vi "Initialize_measurement.vi"(8 "Measurement":string, 9 "Spectrum Only?":bool, 11 "file path":path) -> (0 "error out":errorcluster, 1 "Group Name":string, 3 "tdms file out":refnum<k34>)   [LabVIEW 2019]
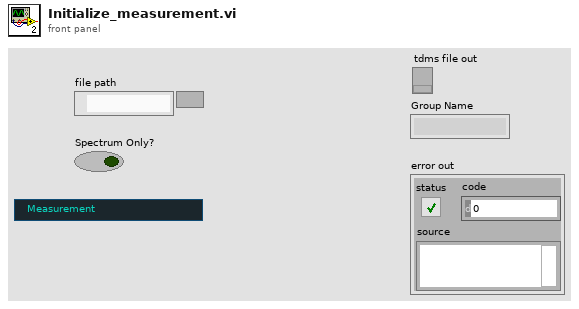
[diagram p1: front panel]
types:
  T1 = enum16{"big-endian, network order", "native, host order", "little-endian"}
  T2 = enum16{"open", "open or create", "create or replace", "create", "open (read-only)"}
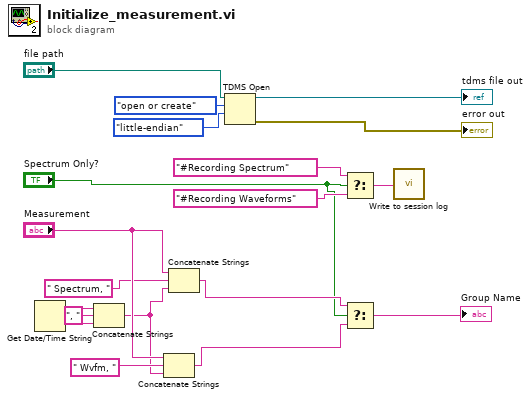
[diagram p0: block diagram]
diagram:
  n1 = Get Date/Time String() -> (date string=w15:string, time string=w13:string)  [unwired: 3 in]
  n2 = Concatenate Strings(w15, ", " ("string"), w13) -> (w14:string)
  n3 = Concatenate Strings("Measurement", " Wvfm, " ("group name in (Untitled)"), w14) -> (w6:string)
  n4 = Concatenate Strings("Measurement", " Spectrum, " ("group name in (Untitled)"), w14) -> (w7:string)
  n5 = TDMS Open(9:T1."little-endian" ("byte order (2:little-endian)"), 10:T2."open or create" ("operation (0:open)"), 11:"file path") -> (0:→"error out":errorcluster, 3:→"tdms file out":refnum<k34>)  [unwired: 4 in]
  n6 = Select(t="#Recording Spectrum" ("Session string"), s="Spectrum Only?", f="#Recording Waveforms" ("Session string")) -> (s? t:f=w8:string)
  n7 = Select(t=w7, s="Spectrum Only?", f=w6) -> (s? t:f=→"Group Name":string)
  n8 = call "Write to session log.vi"("Session string"=w8) -> ()  [unwired: 1 in]
